vi "GetCCDTemperature.vi"(0 "IMAQdx Session In":T2, 1 "错误输入（无错误）":errorcluster) -> (2 "相机温度":T1 {"相机温度 2" scale=0.0..100.0}, 3 "IMAQdx Session Out":T2, 4 "错误输出":errorcluster)   [LabVIEW 2012]
uses:
  <vilib>/userDefined/High Color/IMAQdx.ctl
  <resource>/objmgr/imaqdx.rc
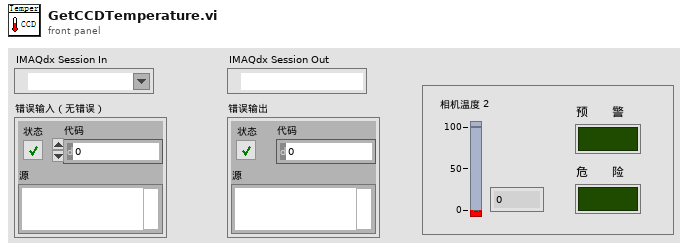
[diagram p1: front panel]
types:
  T1 = cluster{"相机温度 2":dbl, "预      警":bool, "危      险":bool}
  T2 = typedef "IMAQdx.ctl" = refnum<k21>
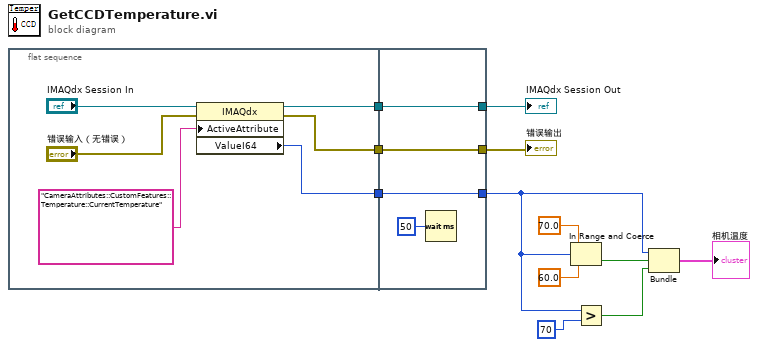
[diagram p0: block diagram]
diagram:
  n1 = flat-sequence {
    tunnel: [w15] -> w11
    tunnel: [w14] -> w10
    tunnel: [w13] -> w8
    tunnel: [w21] -> w12
    tunnel: w11 -> [w21]
    tunnel: [w20] -> w9
    tunnel: w10 -> [w20]
    tunnel: [w19] -> w2
    tunnel: w8 -> [w19]
    frame #0 {
      n2 = property class="IMAQdx"(reference="IMAQdx Session In", error in="错误输入（无错误）", "ActiveAttribute"="CameraAttributes::CustomFeatures::Temperature::CurrentTemperature") -> (reference out=w15:T2, error out=w14:errorcluster, "ValueI64"=w13:i64)
    }
    frame #1 {
      n3 = Wait (ms)(milliseconds to wait=u32 50 ("等待时间（毫秒）")) -> ()  [unwired: 1 out]
    }
  }
  n4 = In Range and Coerce(upper limit=70.0 ("上限"), x=w2, lower limit=60.0 ("下限")) -> (In Range?=w4:bool)  [unwired: 1 out]
  n5 = Greater?(x=w2, y=i64 70) -> (0:w3:bool)
  n6 = Bundle("ValueI64"=w2, w4, w3) -> (→"相机温度":cluster{"ValueI64":i64, bool, bool})  [unwired: 1 in]
  "错误输出" <- w9
  "IMAQdx Session Out" <- w12
